vi "Read Key (Variant)__ogtk.vi"(5 "format string (%;%f)":string="%f", 7 "section":string, 8 "error in (no error)":errorcluster, 9 "type":variant, 10 "key (optional)":string, 11 "refnum":T1) -> (0 "error out":errorcluster, 1 "key-value":variant, 2 "found?":bool, 3 "refnum out":T1)   [LabVIEW 2009]
doc: "Reads a value associated with key in a specified section of the configuration data identified by refnum. If \"key\" input is not specified, the name of the variant object is used as the key. the \"found?\" output will be TRUE for compount objects (clusters) only if all elements (recursively) are found.\n\nFor example a Boolean named \"Enable\" with a value of TRUE would correspond to the key-value pair:\n\nEnable=TRUE\n\nNote: Special characters in section and key names will be escape-coded. These include the following: \\00-\\1F (non-printable chars); \"[\", \"]\", and \"=\" (INI syntax elements); \\FE (\"þ\") and \\FF (\"ÿ\") (legacy bracket encoding); Additionally, the escape character, \"\\\", will be escaped as \"\\\\\"."
uses:
  <vilib>/Utility/config.llb/Config Data RefNum.ctl
  <vilib>/Utility/config.llb/Read Key (I32).vi
  <vilib>/Utility/config.llb/Read Key (U32).vi
  <vilib>/Utility/config.llb/Read Key (Double).vi
  <vilib>/Utility/config.llb/Read Key (String).vi
  <vilib>/Utility/config.llb/Read Key (Boolean).vi
  <vilib>/Utility/config.llb/Read Key (Path).vi
  <vilib>/Utility/config.llb/NI_LVConfig.lvlib
panel:
  in  "Ref for recursive call":refnum<vi>
  # "Read Key (Variant).vi\n\nReads a variant key-value from INI file.\n\nPlease visit http://www.OpenG.org to learn about the\nOpen Source LabVIEW software movement.\n\nNOTICE -- YOU MUST LEAVE THIS NOTICE IN PLACE.  PER THE TERMS OF THE LICENSE BELOW, YOU MAY SUBLICENSE THIS SOFTWARE \nIN ANY WAY THAT DOES NOT CONFLICT WITH THIS LICENSE.\n\n### BSD License (http://www.opensource.org/licenses/bsd-license.php) Begin ###\n \nCopyright (c) 2002, Jean-Pierre Drolet <drolet_jp@hotmail.com>\nCopyright (c) 2002-2006, Jim Kring <jim@jimkring.com>\n\nAll rights reserved.\n\nRedistribution and use in source and binary forms, with or without modification, are permitted provided that the following conditions are met:\n\n    * Redistributions of source code must retain the above copyright notice, this list of conditions and the following disclaimer.\n    * Redistributions in binary form must reproduce the above copyright notice, this list of conditions and the following disclaimer in the \n       documentation and/or other materials provided with the distribution.\n    * Neither the name of SciWare, James Kring, Inc., nor the names of its contributors may be used to endorse or promote products derived \n       from this software without specific prior written permission.\n\nTHIS SOFTWARE IS PROVIDED BY THE COPYRIGHT HOLDERS AND CONTRIBUTORS \"AS IS\" AND ANY EXPRESS OR IMPLIED WARRANTIES, \nINCLUDING, BUT NOT LIMITED TO, THE IMPLIED WARRANTIES OF MERCHANTABILITY AND FITNESS FOR A PARTICULAR PURPOSE ARE \nDISCLAIMED. IN NO EVENT SHALL THE COPYRIGHT OWNER OR CONTRIBUTORS BE LIABLE FOR ANY DIRECT, INDIRECT, INCIDENTAL,\n SPECIAL, EXEMPLARY, OR CONSEQUENTIAL DAMAGES (INCLUDING, BUT NOT LIMITED TO, PROCUREMENT OF SUBSTITUTE GOODS OR \nSERVICES; LOSS OF USE, DATA, OR PROFITS; OR BUSINESS INTERRUPTION) HOWEVER CAUSED AND ON ANY THEORY OF LIABILITY, \nWHETHER IN CONTRACT, STRICT LIABILITY, OR TORT (INCLUDING NEGLIGENCE OR OTHERWISE) ARISING IN ANY WAY OUT OF THE USE \nOF THIS SOFTWARE, EVEN IF ADVISED OF THE POSSIBILITY OF SUCH DAMAGE.\n\n### BSD License End ###"
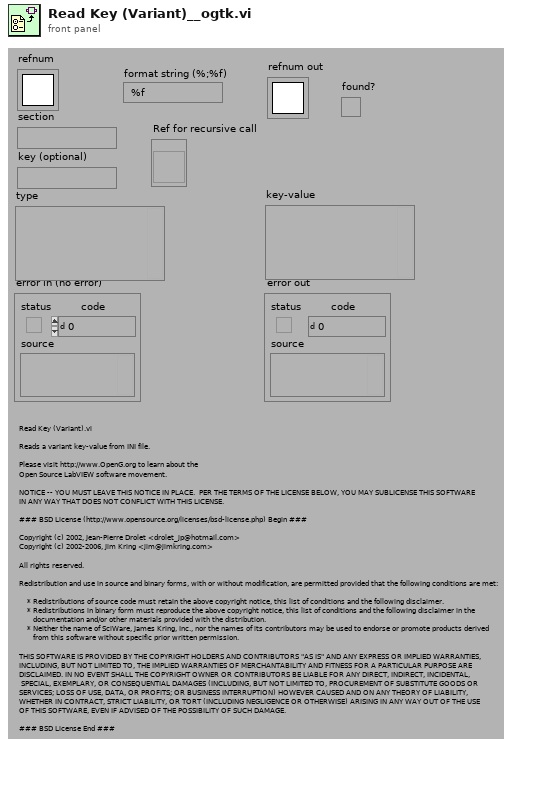
[diagram p1: front panel]
types:
  T1 = typedef "NI_LVConfig.lvlib/Config Data RefNum.ctl" = refnum<k1>
  T2 = typedef "Type Descriptor Enumeration__ogtk.ctl" = enum8{"<Null>", "I8", "I16", "I32", "I64", "U8", "U16", "U32", "U64", "SGL", "DBL", "EXT", "CSG", "CDB", "CXT", "0x0F", "0x10", "0x11", "0x12", "0x13", "0x14", "Enum U8", "Enum U16", "Enum U32", "Enum U64", "SGL PQ", "DBL PQ", "EXT PQ", "CSG PQ", "CDB PQ", "CXT PQ", "0x1F", "0x20", "Boolean", "0x22", "0x23", "0x24", "0x25", "0x26", "0x27", "0x28", "0x29", "0x2A", "0x2B", "0x2C", "0x2D", "0x2E", "0x2F", "String", "0x31", "Path", "Pict", "0x34", "0x35", "0x36", "DAQ", "0x38", "0x39", "0x3A", "0x3B", "0x3C", "0x3D", "0x3E", "0x3F", "Array", "0x41", "0x42", "0x43", "0x44", "0x45", "0x46", "0x47", "0x48", "0x49", "0x4A", "0x4B", "0x4C", "0x4D", "0x4E", "0x4F", "Cluster", "0x51", "0x52", "Variant", "Waveform", "0x55", "0x56", "0x57", "0x58", "0x59", "0x5A", "0x5B", "0x5C", "0x5D", "0x5E", "0x5F", "0x60", "0x61", "0x62", "0x63", "0x64", "0x65", "0x66", "0x67", "0x68", "0x69", "0x6A", "0x6B", "0x6C", "0x6D", "0x6E", "0x6F", "Refnum"}
  T3 = typedef "Type Descriptor__ogtk.ctl" = i16[]
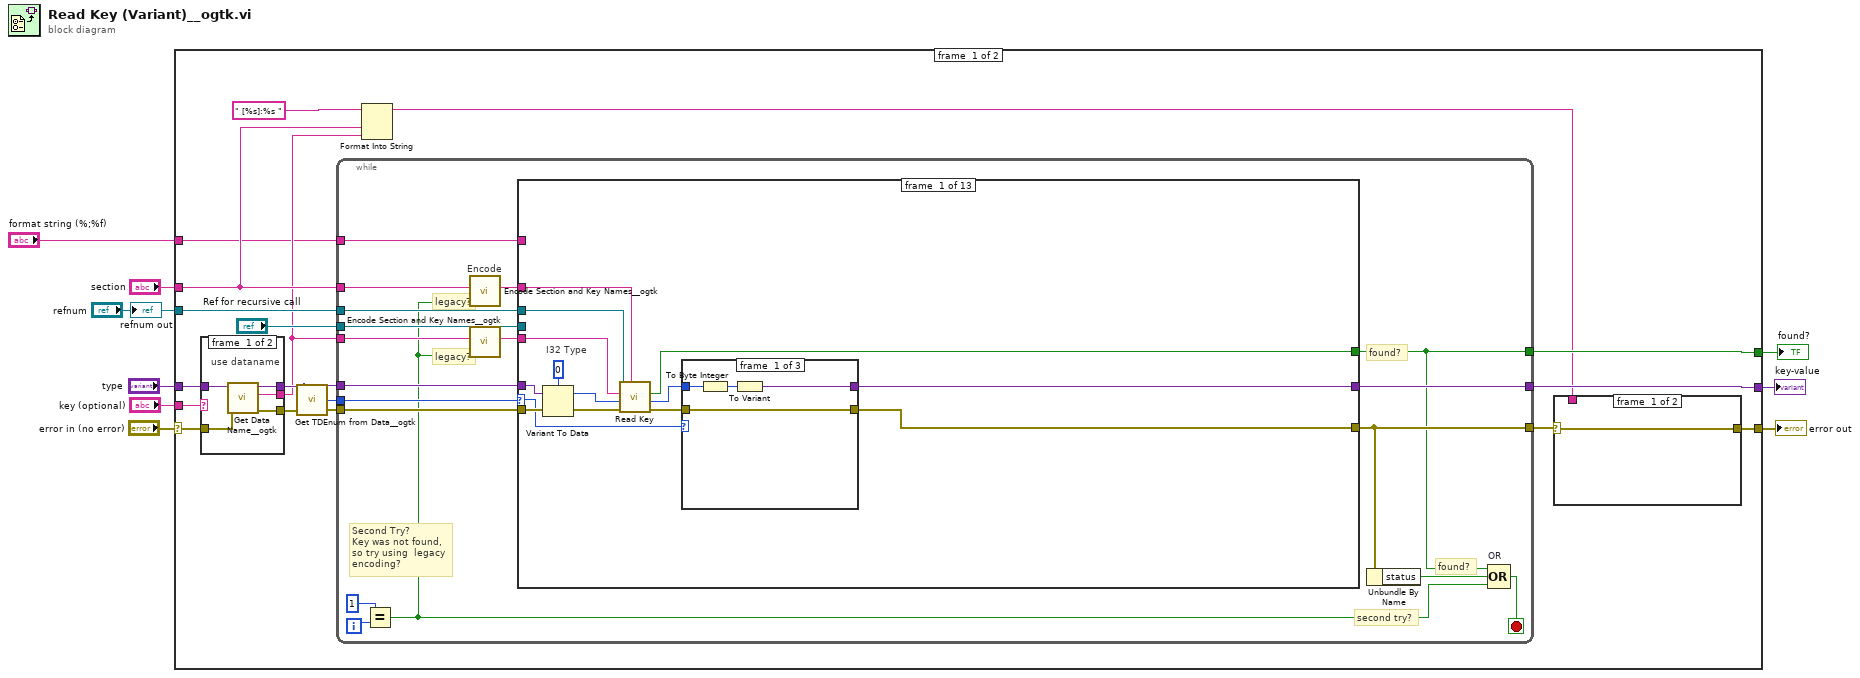
[diagram p0: block diagram]
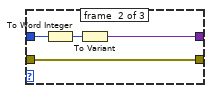
[diagram p2: hidden frame]
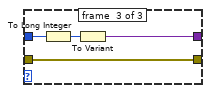
[diagram p3: hidden frame]
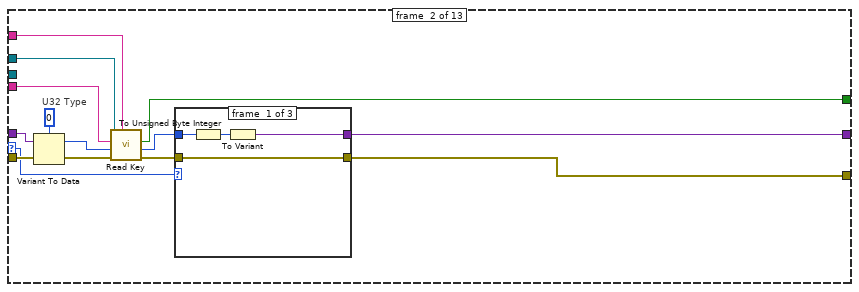
[diagram p4: hidden frame]
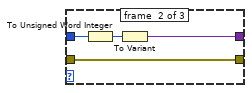
[diagram p5: hidden frame]
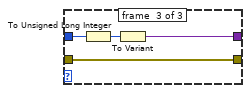
[diagram p6: hidden frame]
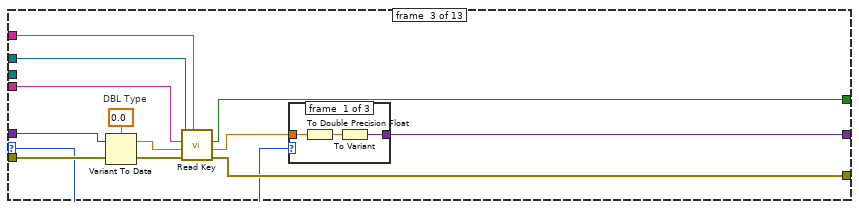
[diagram p7: hidden frame]
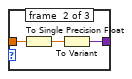
[diagram p8: hidden frame]
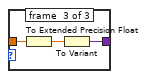
[diagram p9: hidden frame]
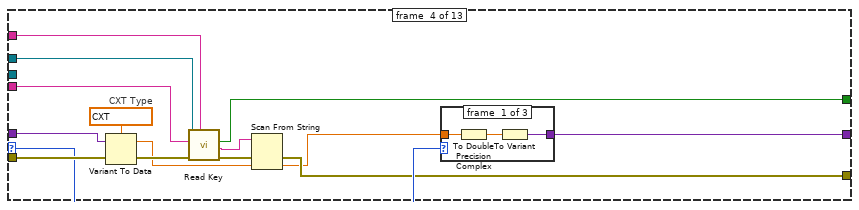
[diagram p10: hidden frame]
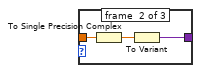
[diagram p11: hidden frame]
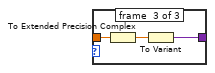
[diagram p12: hidden frame]
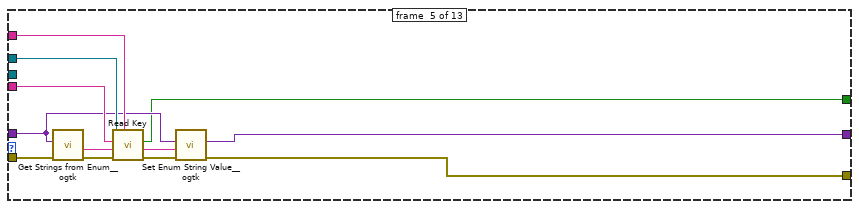
[diagram p13: hidden frame]
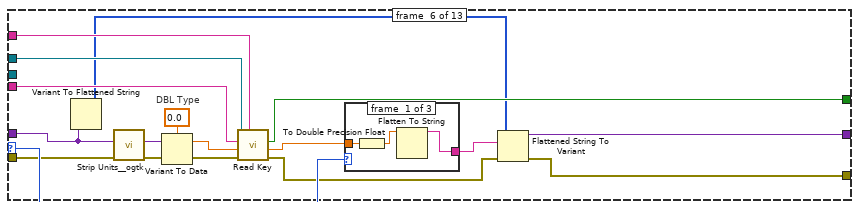
[diagram p14: hidden frame]
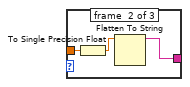
[diagram p15: hidden frame]
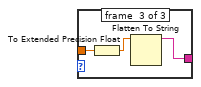
[diagram p16: hidden frame]
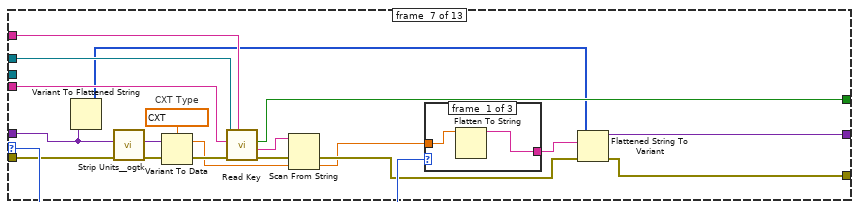
[diagram p17: hidden frame]
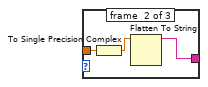
[diagram p18: hidden frame]
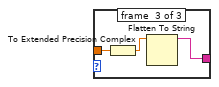
[diagram p19: hidden frame]
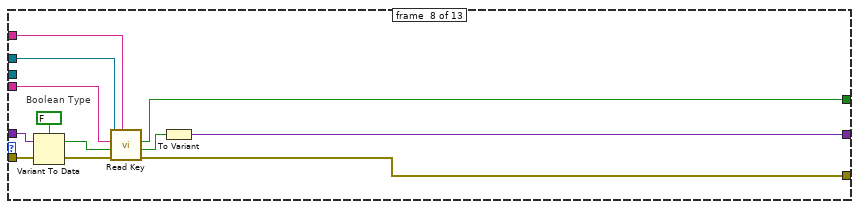
[diagram p20: hidden frame]
diagram:
  n1 = case shown="No Error" "error in (no error)" {
    selector: "error in (no error)" -> [w21 w466]
    tunnel: "refnum" -> [w25 _]
    tunnel: [w15 w466] -> w9
    tunnel: "type" -> [w23 _]
    tunnel: "key (optional)" -> [w22 _]
    tunnel: "section" -> [w12 _]
    tunnel: [w24 variant ("Variant")] -> w4
    tunnel: [w18 FALSE ("found?")] -> w2
    tunnel: "format string (%;%f)" -> [w10 _]
    frame #0 {
      n2 = case shown="\"\"" w22 {
        selector: w22 -> [_ w463]
        tunnel: [w460 w463] -> w11
        tunnel: w23 -> [w457 w461]
        tunnel: w21 -> [w459 w462]
        tunnel: [w458 w462] -> w20
        tunnel: [w456 w461] -> w19
        frame #0 {
          # "use dataname"
          n3 = call "Get Data Name__ogtk.vi"("error in (no error)"=w459, "Data"=w457) -> ("error out"=w458:errorcluster, "Data Name"=w460:string, "Data dup"=w456:variant)  [unwired: 7 in]
        }
        frame #1 {
          # "use optional\nkey"
        }
      }
      n4 = call "Get TDEnum from Data__ogtk.vi"("Data"=w19) -> ("Type Descriptor Enumeration"=w26:T2)  [unwired: 4 in]
      n5 = while {
        tunnel: w26 -> [w44]
        tunnel: w25 -> [w43]
        tunnel: [w42] -> w24
        tunnel: w20 -> [w41]
        tunnel: w19 -> [w40]
        tunnel: [w32] -> w18
        tunnel: "Ref for recursive call" -> [w39]
        tunnel: [w34] -> w16
        tunnel: w12 -> [w37]
        tunnel: w11 -> [w36]
        tunnel: w10 -> [w27]
        i -> [w31]
        stop <- w29 stop-if-true
        # "found?"
        # "found?"
        # "second try?"
        # "legacy?"
        # "legacy?"
        # "Second Try?\nKey was not found, so try using  legacy encoding?"
        # "Encode"
        n6 = Equal?(x=1, y=w31) -> (x = y?=w28:bool)
        n7 = call "Encode Section and Key Names__ogtk.vi"("use legacy encoding scheme? (FALSE)"=w28, "string"=w37) -> ("encoded string"=w38:string)  [unwired: 9 in]
        n8 = call "Encode Section and Key Names__ogtk.vi"("use legacy encoding scheme? (FALSE)"=w28, "string"=w36) -> ("encoded string"=w35:string)  [unwired: 9 in]
        n9 = case shown="\"Array\"" w44 {
          selector: w44 -> [w47 w73 w97 w124 _ w164 w195 _ _ _ _ _ _]
          tunnel: w40 -> [w57 w83 w108 w132 w145 w157 w189 w220 w232 w244 w248 w396 w446]
          tunnel: w43 -> [w56 w82 w107 w131 w154 w171 w200 w219 w231 w243 w255 w410 w449]
          tunnel: [w46 w71 w105 w122 w147 w159 w191 w217 w229 w241 w252 w399 w440] -> w34
          tunnel: w41 -> [w54 w80 w104 w129 w151 w163 w194 w216 w228 w240 w258 w398 w442]
          tunnel: w35 -> [w53 w79 w103 w128 w153 w169 w198 w215 w227 w239 w249 w408 w448]
          tunnel: w38 -> [w52 w78 w102 w127 w152 w168 w197 w214 w226 w238 w250 w409 w447]
          tunnel: [w45 w75 w99 w126 w144 w155 w187 w211 w225 w235 w253 w400 w443] -> w42
          tunnel: [w50 w74 w98 w125 w143 w165 w196 w210 w222 w234 w251 w404 w438] -> w32
          tunnel: w39 -> [_ _ _ _ _ _ _ _ _ _ w254 w403 _]
          tunnel: w27 -> [_ _ _ _ _ _ _ _ _ _ w246 w393 _]
          frame #0 {
            # "I32 Type"
            n10 = Variant To Data(error in=w54, Variant=w57, type=0) -> (error out=w55:errorcluster, data=w51:i32)
            n11 = call-poly <vilib>:"Read Key.vi"("section"=w52, "error in (no error)"=w55, "default value"=w51, "key"=w53, "refnum"=w56) -> ("error out"=w49:errorcluster, "value"=w48:i32, "found?"=w50:bool)  [unwired: 3 in, 1 out]
            n12 = case shown="\"I32\", Default" w47 {
              tunnel: w48 -> [w62 w66 w70]
              tunnel: [w61 w65 w69] -> w45
              tunnel: w49 -> [w59 w63 w67]
              tunnel: [w59 w63 w67] -> w46
              frame #0 {
                n13 = To Byte Integer(number=w62) -> (8bit integer=w60:i8)
                n14 = To Variant(anything=w60) -> (Variant=w61:variant)
              }
              frame #1 {
                n15 = To Word Integer(number=w66) -> (16bit integer=w64:i16)
                n16 = To Variant(anything=w64) -> (Variant=w65:variant)
              }
              frame #2 {
                n17 = To Long Integer(number=w70) -> (32bit integer=w68:i32)
                n18 = To Variant(anything=w68) -> (Variant=w69:variant)
              }
            }
          }
          frame #1 {
            # "U32 Type"
            n19 = Variant To Data(error in=w80, Variant=w83, type=u32 0) -> (error out=w81:errorcluster, data=w77:u32)
            n20 = call-poly <vilib>:"Read Key.vi"("section"=w78, "error in (no error)"=w81, "default value"=w77, "key"=w79, "refnum"=w82) -> ("error out"=w72:errorcluster, "value"=w76:u32, "found?"=w74:bool)  [unwired: 3 in, 1 out]
            n21 = case shown="\"U32\", Default" w73 {
              tunnel: w76 -> [w88 w92 w96]
              tunnel: [w87 w91 w95] -> w75
              tunnel: w72 -> [w85 w89 w93]
              tunnel: [w85 w89 w93] -> w71
              frame #0 {
                n22 = To Unsigned Byte Integer(number=w88) -> (unsigned 8bit integer=w86:u8)
                n23 = To Variant(anything=w86) -> (Variant=w87:variant)
              }
              frame #1 {
                n24 = To Unsigned Word Integer(number=w92) -> (unsigned 16bit integer=w90:u16)
                n25 = To Variant(anything=w90) -> (Variant=w91:variant)
              }
              frame #2 {
                n26 = To Unsigned Long Integer(number=w96) -> (unsigned 32bit integer=w94:u32)
                n27 = To Variant(anything=w94) -> (Variant=w95:variant)
              }
            }
          }
          frame #2 {
            # "DBL Type"
            n28 = Variant To Data(error in=w104, Variant=w108, type=0.0) -> (error out=w106:errorcluster, data=w101:dbl)
            n29 = call-poly <vilib>:"Read Key.vi"("section"=w102, "error in (no error)"=w106, "default value"=w101, "key"=w103, "refnum"=w107) -> ("error out"=w105:errorcluster, "value"=w100:dbl, "found?"=w98:bool)  [unwired: 3 in, 1 out]
            n30 = case shown="\"DBL\", Default" w97 {
              tunnel: w100 -> [w112 w115 w118]
              tunnel: [w111 w114 w117] -> w99
              frame #0 {
                n31 = To Double Precision Float(number=w112) -> (double precision float=w110:dbl)
                n32 = To Variant(anything=w110) -> (Variant=w111:variant)
              }
              frame #1 {
                n33 = To Single Precision Float(number=w115) -> (single precision float=w113:sgl)
                n34 = To Variant(anything=w113) -> (Variant=w114:variant)
              }
              frame #2 {
                n35 = To Extended Precision Float(1:w118) -> (0:w116:ext)
                n36 = To Variant(anything=w116) -> (Variant=w117:variant)
              }
            }
          }
          frame #3 {
            # "CXT Type"
            n37 = Variant To Data(error in=w129, Variant=w132, type=cxt 0.0+0.0i) -> (error out=w130:errorcluster, data=w120:cxt)
            n38 = call-poly <vilib>:"Read Key.vi"("section"=w127, "error in (no error)"=w130, "key"=w128, "refnum"=w131) -> ("error out"=w123:errorcluster, "value"=w121:string, "found?"=w125:bool)  [unwired: 4 in, 1 out]
            n39 = Scan From String(input string=w121, error in=w123, default 1=w120) -> (error out=w122:errorcluster, output 1=w119:cxt)  [unwired: 2 in, 2 out]
            n40 = case shown="\"CDB\", Default" w124 {
              tunnel: w119 -> [w136 w139 w142]
              tunnel: [w135 w138 w141] -> w126
              frame #0 {
                n41 = To Double Precision Complex(1:w136) -> (0:w134:cdb)
                n42 = To Variant(anything=w134) -> (Variant=w135:variant)
              }
              frame #1 {
                n43 = To Single Precision Complex(1:w139) -> (0:w137:csg)
                n44 = To Variant(anything=w137) -> (Variant=w138:variant)
              }
              frame #2 {
                n45 = To Extended Precision Complex(1:w142) -> (0:w140:cxt)
                n46 = To Variant(anything=w140) -> (Variant=w141:variant)
              }
            }
          }
          frame #4 {
            n47 = call "Get Strings from Enum__ogtk.vi"("error in (no error)"=w151, "Enum"=w145) -> ("error out"=w150:errorcluster, "String Value"=w149:string)  [unwired: 6 in, 2 out]
            n48 = call-poly <vilib>:"Read Key.vi"("section"=w152, "error in (no error)"=w150, "default value"=w149, "key"=w153, "refnum"=w154) -> ("error out"=w148:errorcluster, "value"=w146:string, "found?"=w143:bool)  [unwired: 3 in, 1 out]
            n49 = call "Set Enum String Value__ogtk.vi"("error in (no error)"=w148, "String Value"=w146, "Default Enum Value"=w145) -> ("error out"=w147:errorcluster, "Enum"=w144:variant)  [unwired: 7 in]
          }
          frame #5 {
            # "DBL Type"
            n50 = Variant To Flattened String(Variant=w157) -> (1:w156:i16[])  [unwired: 1 out]
            n51 = call "Strip Units__ogtk.vi"("error in (no error)"=w163, "Number or 1D array with units"=w157) -> ("error out"=w161:errorcluster, "Pure Number(s) (base units)"=w162:variant)  [unwired: 8 in]
            n52 = Variant To Data(error in=w161, Variant=w162, type=0.0) -> (error out=w170:errorcluster, data=w167:dbl)
            n53 = call-poly <vilib>:"Read Key.vi"("section"=w168, "error in (no error)"=w170, "default value"=w167, "key"=w169, "refnum"=w171) -> ("error out"=w160:errorcluster, "value"=w166:dbl, "found?"=w165:bool)  [unwired: 3 in, 1 out]
            n54 = case shown="\"DBL PQ\", Default" w164 {
              tunnel: w166 -> [w175 w178 w181]
              tunnel: [w174 w176 w179] -> w158
              frame #0 {
                n55 = To Double Precision Float(number=w175) -> (double precision float=w173:dbl)
                n56 = Flatten To String(anything=w173) -> (data string=w174:string)  [unwired: 3 in, 2 out]
              }
              frame #1 {
                n57 = To Single Precision Float(number=w178) -> (single precision float=w177:sgl)
                n58 = Flatten To String(anything=w177) -> (data string=w176:string)  [unwired: 3 in, 2 out]
              }
              frame #2 {
                n59 = To Extended Precision Float(1:w181) -> (0:w180:ext)
                n60 = Flatten To String(anything=w180) -> (data string=w179:string)  [unwired: 3 in, 2 out]
              }
            }
            n61 = Flattened String To Variant(4:w160, 6:w158, 7:w156) -> (0:w159:errorcluster, 3:w155:variant)
          }
          frame #6 {
            # "CXT Type"
            n62 = Variant To Flattened String(Variant=w189) -> (1:w188:i16[])  [unwired: 1 out]
            n63 = call "Strip Units__ogtk.vi"("error in (no error)"=w194, "Number or 1D array with units"=w189) -> ("error out"=w192:errorcluster, "Pure Number(s) (base units)"=w193:variant)  [unwired: 8 in]
            n64 = Variant To Data(error in=w192, Variant=w193, type=cxt 0.0+0.0i) -> (error out=w199:errorcluster, data=w183:cxt)
            n65 = call-poly <vilib>:"Read Key.vi"("section"=w197, "error in (no error)"=w199, "key"=w198, "refnum"=w200) -> ("error out"=w185:errorcluster, "value"=w184:string, "found?"=w196:bool)  [unwired: 4 in, 1 out]
            n66 = Scan From String(input string=w184, error in=w185, default 1=w183) -> (error out=w186:errorcluster, output 1=w182:cxt)  [unwired: 2 in, 2 out]
            n67 = case shown="\"CDB PQ\", Default" w195 {
              tunnel: w182 -> [w203 w206 w209]
              tunnel: [w202 w204 w207] -> w190
              frame #0 {
                n68 = Flatten To String(anything=w203) -> (data string=w202:string)  [unwired: 3 in, 2 out]
              }
              frame #1 {
                n69 = To Single Precision Complex(1:w206) -> (0:w205:csg)
                n70 = Flatten To String(anything=w205) -> (data string=w204:string)  [unwired: 3 in, 2 out]
              }
              frame #2 {
                n71 = To Extended Precision Complex(1:w209) -> (0:w208:cxt)
                n72 = Flatten To String(anything=w208) -> (data string=w207:string)  [unwired: 3 in, 2 out]
              }
            }
            n73 = Flattened String To Variant(4:w186, 6:w190, 7:w188) -> (0:w191:errorcluster, 3:w187:variant)
          }
          frame #7 {
            # "Boolean Type"
            n74 = Variant To Data(error in=w216, Variant=w220, type=FALSE) -> (error out=w218:errorcluster, data=w213:bool)
            n75 = call-poly <vilib>:"Read Key.vi"("section"=w214, "error in (no error)"=w218, "default value"=w213, "key"=w215, "refnum"=w219) -> ("error out"=w217:errorcluster, "value"=w212:bool, "found?"=w210:bool)  [unwired: 3 in, 1 out]
            n76 = To Variant(anything=w212) -> (Variant=w211:variant)
          }
          frame #8 {
            # "String Type"
            n77 = Variant To Data(error in=w228, Variant=w232, type="") -> (error out=w230:errorcluster, data=w223:string)
            n78 = call-poly <vilib>:"Read Key.vi"("section"=w226, "error in (no error)"=w230, "default value"=w223, "key"=w227, "refnum"=w231) -> ("error out"=w229:errorcluster, "value"=w224:string, "found?"=w222:bool)  [unwired: 3 in, 1 out]
            n79 = To Variant(anything=w224) -> (Variant=w225:variant)
          }
          frame #9 {
            # "Path Type"
            n80 = Variant To Data(error in=w240, Variant=w244, type=path "") -> (error out=w242:errorcluster, data=w237:path)
            n81 = call-poly <vilib>:"Read Key.vi"("section"=w238, "error in (no error)"=w242, "default value"=w237, "key"=w239, "refnum"=w243) -> ("error out"=w241:errorcluster, "value"=w236:path, "found?"=w234:bool)  [unwired: 3 in, 1 out]
            n82 = To Variant(anything=w236) -> (Variant=w235:variant)
          }
          frame #10 {
            n83 = call "Reshape Array to 1D VArray__ogtk.vi"("error in (no error)"=w258, "MultiD Array"=w248) -> ("error out"=w259:errorcluster, "1D VArray"=w247:variant)  [unwired: 7 in, 1 out]
            n84 = call "Get Array Element TDEnum__ogtk.vi"("error in (no error)"=w259, "Array"=w247) -> ("error out"=w256:errorcluster, "Element Type"=w257:T2)  [unwired: 8 in]
            n85 = case shown="Default" w257 {
              selector: w257 -> [_ w339]
              tunnel: w256 -> [_ w349]
              tunnel: w248 -> [w269 w327]
              tunnel: w250 -> [w267 w350]
              tunnel: w255 -> [w266 w351]
              tunnel: w249 -> [w270 w352]
              tunnel: w254 -> [w268 _]
              tunnel: [w264 w326] -> w253
              tunnel: [w263 errorcluster {"status"=FALSE, "code"=0, "source"=""} ("error out")] -> w252
              tunnel: [w262 w348] -> w251
              tunnel: w246 -> [w260 w324]
              frame #0 {
                n86 = Concatenate Strings(w270, ".<size(s)>" ("Substring")) -> (w273:string)
                n87 = call-poly <vilib>:"Read Key.vi"("read raw string? (F)"=TRUE, "section"=w267, "key"=w273, "refnum"=w266) -> ("error out"=w271:errorcluster, "value"=w272:string, "found?"=w261:bool)  [unwired: 4 in, 1 out]
                n88 = case shown="True" w261 {
                  tunnel: w272 -> [_ w304]
                  tunnel: w271 -> [_ w280]
                  tunnel: w270 -> [_ w299]
                  tunnel: w269 -> [w276 w298]
                  tunnel: w268 -> [_ w297]
                  tunnel: w267 -> [_ w295]
                  tunnel: w266 -> [_ w294]
                  tunnel: [w276 w287] -> w264
                  tunnel: [errorcluster {"status"=FALSE, "code"=0, "source"=""} ("error out") w286] -> w263
                  tunnel: [FALSE w284] -> w262
                  tunnel: w260 -> [_ w278]
                  frame #0 {
                    # "array size(s) not found. Ignore element keys (if any) and return input array"
                  }
                  frame #1 {
                    # "array.size(s) is found. Read elements keys. missing keys replace with datatype default."
                    n89 = call "Get Array Element TD__ogtk.vi"("error in (no error)"=w280, "Array"=w298) -> ("error out"=w282:errorcluster, "Type Descriptor"=w283:T3)  [unwired: 8 in]
                    n90 = property class="VI"() -> ("VI Name"=w301:string)  [unwired: 2 in, 2 out]
                    n91 = call "Get Default Data from TD__ogtk.vi"("error in (no error)"=w282, "Type Descriptor"=w283) -> ("error out"=w279:errorcluster, "Default VData"=w281:variant)  [unwired: 8 in]
                    n92 = Spreadsheet String To Array(delimiter (Tab)=" ", format string="%d", spreadsheet string=w304, array type (2D Dbl)=u32[] [] ("Array Constant")) -> (array=w288:u32[])
                    n93 = Open VI Reference(type specifier VI Refnum (for type only)=w297, vi path=w301, error in (no error)=w279) -> (vi reference=w296:refnum<vi>, error out=w300:errorcluster)  [unwired: 3 in]
                    n94 = Multiply Array Elements(1:w288) -> (0:w302:u32)
                    n95 = for {
                      N: w302 -> [_]
                      shift-right: [w317] -> w291
                      shift-left: w300 -> [w314]
                      shift-right: [w318] -> w293
                      shift-left: w296 -> [w316]
                      tunnel: w299 -> [w321]
                      tunnel: w281 -> [w315]
                      tunnel: w295 -> [w312]
                      tunnel: w294 -> [w311]
                      tunnel: [w310] -> w292 mode=indexing
                      tunnel: [w309] -> w285 mode=indexing
                      tunnel: w278 -> [w308]
                      i -> [w322]
                      n96 = Format Into String(format string=" %d" ("Format String"), initial string=w321, w322) -> (resulting string=w313:string)  [unwired: 1 in, 1 out]
                      n97 = call-by-ref "?"(reference=w316, error in=w314, "format string (%;%f"=w308, "section"=w312, "type"=w315, "key (optional)"=w313, "refnum"=w311) -> (reference out=w318:refnum<vi>, error out=w320:errorcluster, "error out"=w319:errorcluster, "key-value"=w310:variant, "found?"=w309:bool)  [unwired: 3 in, 1 out]
                      n98 = Build Array(w320, w319) -> (w307:errorcluster[])
                      n99 = call <vilib>:"Merge Errors.vi"("error array in"=w307) -> ("error out"=w317:errorcluster)  [unwired: 6 in]
                    }
                    n100 = And Array Elements(Boolean array=w285) -> (logical AND=w284:bool)
                    n101 = Close Reference(reference=w293) -> ()  [unwired: 1 in, 1 out]
                    n102 = call "Array of VData to VArray__ogtk.vi"("error in (no error)"=w291, "Element Type (when empty)"=w281, "1D Array of VData"=w292) -> ("error out"=w290:errorcluster, "VArray"=w289:variant)  [unwired: 7 in]
                    n103 = call "Reshape 1D Array__ogtk.vi"("error in (no error)"=w290, "Size(s)"=w288, "1D Array"=w289) -> ("error out"=w286:errorcluster, "Reshaped VArray"=w287:variant)  [unwired: 7 in]
                  }
                }
              }
              frame #1 {
                n104 = call-poly <vilib>:"Read Key.vi"("section"=w350, "error in (no error)"=w349, "key"=w352, "refnum"=w351) -> ("error out"=w347:errorcluster, "value"=w353:string, "found?"=w348:bool)  [unwired: 4 in, 1 out]
                n105 = Scan From String(format string="<size(s)=%[\\s0-9]> " ("regular expression"), input string=w353, error in=w347) -> (remaining string=w340:string, error out=w330:errorcluster, output 1=w345:string)  [unwired: 2 in, 1 out]
                n106 = Variant To Flattened String(Variant=w327) -> (data string=w332:string, 1:w333:i16[])
                n107 = Spreadsheet String To Array(delimiter (Tab)=" ", format string="%d", spreadsheet string=w345, array type (2D Dbl)=u32[] []) -> (array=w346:u32[])
                n108 = Type Cast(x=w346) -> (*(type *) &x=w337:string)  [unwired: 1 in]
                n109 = Spreadsheet String To Array(delimiter (Tab)=" ", format string=w324, spreadsheet string=w340, array type (2D Dbl)=dbl[] []) -> (array=w338:dbl[])
                n110 = case shown="\"SGL\", \"SGL PQ\"" w339 {
                  tunnel: w338 -> [_ w360 w364 w368 w372 w376 w380 w384 w386 w390]
                  tunnel: [w355 w358 w362 w366 w370 w374 w378 w382 w388 w392] -> w335
                  tunnel: ["" w357 w361 w365 w369 w373 w377 w381 w387 w391] -> w334
                  tunnel: w337 -> [_ w357 w361 w365 w369 w373 w377 w381 w387 w391]
                  tunnel: w332 -> [w355 _ _ _ _ _ _ _ _ _]
                  frame #0 {
                  }
                  frame #1 {
                    n111 = To Byte Integer(number=w360) -> (8bit integer=w359:i8[])
                    n112 = Type Cast(x=w359) -> (*(type *) &x=w358:string)  [unwired: 1 in]
                  }
                  frame #2 {
                    n113 = To Word Integer(number=w364) -> (16bit integer=w363:i16[])
                    n114 = Type Cast(x=w363) -> (*(type *) &x=w362:string)  [unwired: 1 in]
                  }
                  frame #3 {
                    n115 = To Long Integer(number=w368) -> (32bit integer=w367:i32[])
                    n116 = Type Cast(x=w367) -> (*(type *) &x=w366:string)  [unwired: 1 in]
                  }
                  frame #4 {
                    n117 = To Unsigned Byte Integer(number=w372) -> (unsigned 8bit integer=w371:u8[])
                    n118 = Type Cast(x=w371) -> (*(type *) &x=w370:string)  [unwired: 1 in]
                  }
                  frame #5 {
                    n119 = To Unsigned Word Integer(number=w376) -> (unsigned 16bit integer=w375:u16[])
                    n120 = Type Cast(x=w375) -> (*(type *) &x=w374:string)  [unwired: 1 in]
                  }
                  frame #6 {
                    n121 = To Unsigned Long Integer(number=w380) -> (unsigned 32bit integer=w379:u32[])
                    n122 = Type Cast(x=w379) -> (*(type *) &x=w378:string)  [unwired: 1 in]
                  }
                  frame #7 {
                    n123 = To Single Precision Float(number=w384) -> (single precision float=w383:sgl[])
                    n124 = Type Cast(x=w383) -> (*(type *) &x=w382:string)  [unwired: 1 in]
                  }
                  frame #8 {
                    n125 = To Double Precision Float(number=w386) -> (double precision float=w385:dbl[])
                    n126 = Type Cast(x=w385) -> (*(type *) &x=w388:string)  [unwired: 1 in]
                  }
                  frame #9 {
                    n127 = To Extended Precision Float(1:w390) -> (0:w389:ext[])
                    n128 = Type Cast(x=w389) -> (*(type *) &x=w392:string)  [unwired: 1 in]
                  }
                }
                n129 = Concatenate Strings(w334, w335) -> (w336:string)
                n130 = Flattened String To Variant(4:w330, 6:w336, 7:w333) -> (0:w329:errorcluster, 3:w328:variant)
                n131 = Select(t=w327, s=w329, f=w328) -> (s? t:f=w326:variant)
              }
            }
          }
          frame #11 {
            # ">> Cluster Name >>"
            # "Expand cluster to its elements\nand read keys recursively."
            n132 = call "Get Data Name__ogtk.vi"("error in (no error)"=w398, "Data"=w396) -> ("error out"=w397:errorcluster, "Data Name"=w394:string, "Data dup"=w395:variant)  [unwired: 7 in]
            n133 = call "Cluster to Array of VData__ogtk.vi"("error in (no error)"=w397, "Cluster"=w395) -> ("error out"=w416:errorcluster, "Array of VData"=w415:variant[])  [unwired: 8 in]
            n134 = property class="VI"() -> ("VI Name"=w414:string)  [unwired: 2 in, 2 out]
            n135 = Open VI Reference(type specifier VI Refnum (for type only)=w403, vi path=w414, error in (no error)=w416) -> (vi reference=w411:refnum<vi>, error out=w413:errorcluster)  [unwired: 3 in]
            n136 = for {
              shift-right: [w436] -> w412
              shift-left: w411 -> [w437]
              shift-right: [w421] -> w406
              shift-left: w413 -> [w432]
              tunnel: w415 -> [w430] mode=indexing
              tunnel: w409 -> [w426]
              tunnel: w410 -> [w427]
              tunnel: w408 -> [w434]
              tunnel: [w423] -> w407 mode=indexing
              tunnel: [w419] -> w405 mode=indexing
              tunnel: w393 -> [w418]
              n137 = call "Get Data Name__ogtk.vi"("error in (no error)"=w432, "Data"=w430) -> ("error out"=w431:errorcluster, "Data Name"=w420:string, "Data dup"=w429:variant)  [unwired: 7 in]
              n138 = Format Into String(format string=".%s" ("Format String"), initial string=w434, w420) -> (resulting string=w428:string)  [unwired: 1 in, 1 out]
              n139 = call-by-ref "?"(reference=w437, error in=w431, "format string (%;%f"=w418, "section"=w426, "type"=w429, "key (optional)"=w428, "refnum"=w427) -> (reference out=w436:refnum<vi>, error out=w435:errorcluster, "error out"=w425:errorcluster, "key-value"=w424:variant, "found?"=w419:bool)  [unwired: 3 in, 1 out]
              n140 = Build Array(w435, w425) -> (w417:errorcluster[])
              n141 = call <vilib>:"Merge Errors.vi"("error array in"=w417) -> ("error out"=w422:errorcluster)  [unwired: 6 in]
              n142 = call "Set Data Name__ogtk.vi"("error in (no error)"=w422, "Data Name"=w420, "Data"=w424) -> ("error out"=w421:errorcluster, "Renamed Data"=w423:variant)  [unwired: 7 in]
            }
            n143 = And Array Elements(Boolean array=w405) -> (logical AND=w404:bool)
            n144 = call "Array of VData to VCluster__ogtk.vi"("error in (no error)"=w406, "Array"=w407) -> ("error out"=w402:errorcluster, "VCluster"=w401:variant)  [unwired: 8 in]
            n145 = Close Reference(reference=w412) -> ()  [unwired: 1 in, 1 out]
            n146 = call "Set Data Name__ogtk.vi"("error in (no error)"=w402, "Data Name"=w394, "Data"=w401) -> ("error out"=w399:errorcluster, "Renamed Data"=w400:variant)  [unwired: 7 in]
          }
          frame #12 {
            n147 = Variant To Flattened String(Variant=w446) -> (data string=w445:string, 1:w439:i16[])
            n148 = call-poly <vilib>:"Read Key.vi"("section"=w447, "error in (no error)"=w442, "default value"=w445, "key"=w448, "refnum"=w449) -> ("error out"=w441:errorcluster, "value"=w444:string, "found?"=w438:bool)  [unwired: 3 in, 1 out]
            n149 = Flattened String To Variant(4:w441, 6:w444, 7:w439) -> (0:w440:errorcluster, 3:w443:variant)
          }
        }
        n150 = Unbundle By Name(w34) -> ("status"=w33:bool)
        n151 = Compound Arithmetic op=OR "OR"(w32, w33, w28) -> (w29:bool)
      }
      n152 = Format Into String(format string=" [%s]:%s " ("Format String"), w12, w11) -> (resulting string=w13:string)  [unwired: 2 in, 1 out]
      n153 = case shown="Error" w16 {
        selector: w16 -> [w450 w455]
        tunnel: [w450 w454] -> w15
        tunnel: w13 -> [_ w451]
        frame #0 {
        }
        frame #1 {
          # "Add section and key names to\nerror source."
          n154 = Unbundle By Name(w455) -> ("source"=w452:string)
          n155 = Concatenate Strings(w451, w452) -> (w453:string)
          n156 = Bundle By Name(cluster=w455, "source"=w453) -> (w454:errorcluster)
        }
      }
    }
    frame #1 {
    }
  }
  "error out" <- w9
  "key-value" <- w4
  "found?" <- w2
  "refnum out" <- "refnum"
